vi "Average.vi"() -> ()   [LabVIEW 2020]
panel:
  out "Average":dbl
  in  "X5":dbl
  in  "X4":dbl
  in  "X3":dbl
  in  "X2":dbl
  in  "X1":dbl
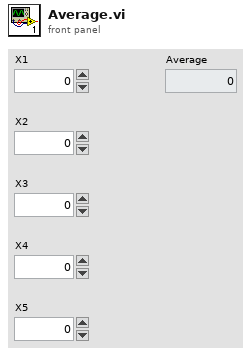
[diagram p1: front panel]
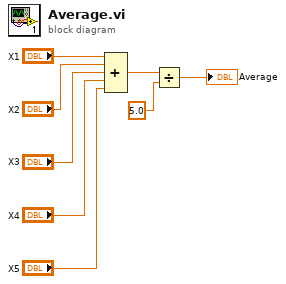
[diagram p0: block diagram]
diagram:
  n1 = Compound Arithmetic op=ADD("X1", "X2", "X3", "X4", "X5") -> (w3:dbl)
  n2 = Divide(x=w3, y=5.0) -> (x/y=→"Average":dbl)
